vi "users Template Keys.vi"(6 "Current User Record":T1, 7 "Edit sxUsername (\"\")":string, 8 "error in (no error)":errorcluster, 9 "Copy? (f)":bool, 10 "Edit? (f)":bool, 11 "Connection Refnum":T2) -> (0 "error out":errorcluster, 1 "Template Keys":T3, 3 "Connection Refnum":T2)   [LabVIEW 2011]
uses:
  ITK EXT/utils/keyedarr.llb/Keyed Array.ctl
  Summitek EXT/ODBC/SQL Controls/Connection Refnum.ctl
  server/database/Users/User Record.ctl
  ITK EXT/utils/strutil.llb/Case Matching.ctl
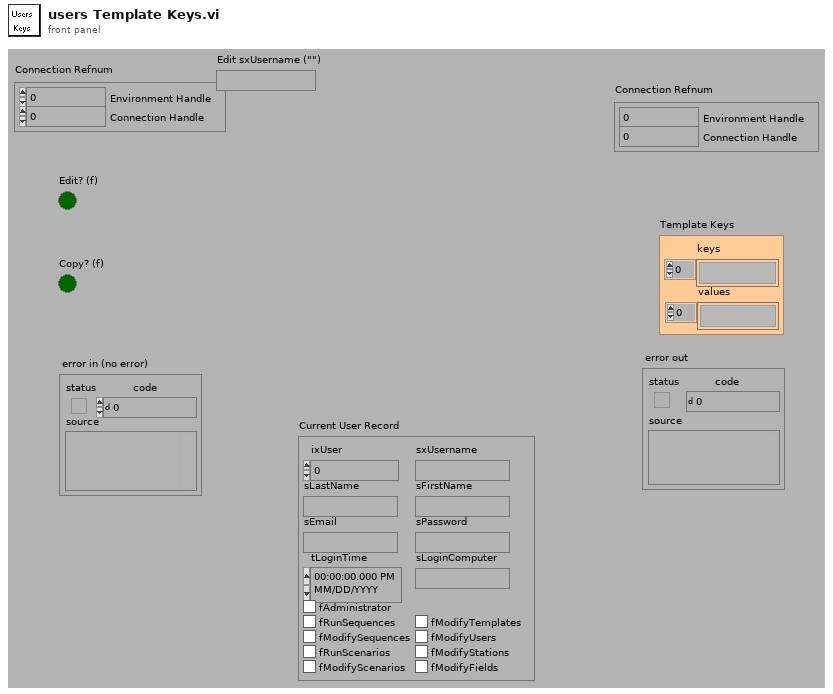
[diagram p1: front panel]
types:
  T1 = typedef "User Record.ctl" = cluster{"ixUser":i32, "sxUsername":string, "sLastName":string, "sFirstName":string, "sEmail":string, "sPassword":string, "tLoginTime":timestamp, "sLoginComputer":string, "fAdministrator":bool, "fRunSequences":bool, "fModifySequences":bool, "fRunScenarios":bool, "fModifyScenarios":bool, "fModifyTemplates":bool, "fModifyUsers":bool, "fModifyStations":bool, "fModifyFields":bool}
  T2 = typedef "Connection Refnum.ctl" = cluster{"Environment Handle":i32, "Connection Handle":i32}
  T3 = typedef "Keyed Array.ctl" = cluster{"keys":string[], "values":string[]}
  T4 = typedef "Authorization Data.ctl" = cluster{"Valid":bool, "Seats":i32, "Expire Time":timestamp, "Last Access Time":timestamp, "Product ID":string, "Hardware ID":string, "Spartan Serial Number":string, "Feature":cluster{"#attributes":cluster{"Name":string, "Value":string}}[]}
  T5 = typedef "Case Matching.ctl" = enum16{"a != A", "a == A", "system"}
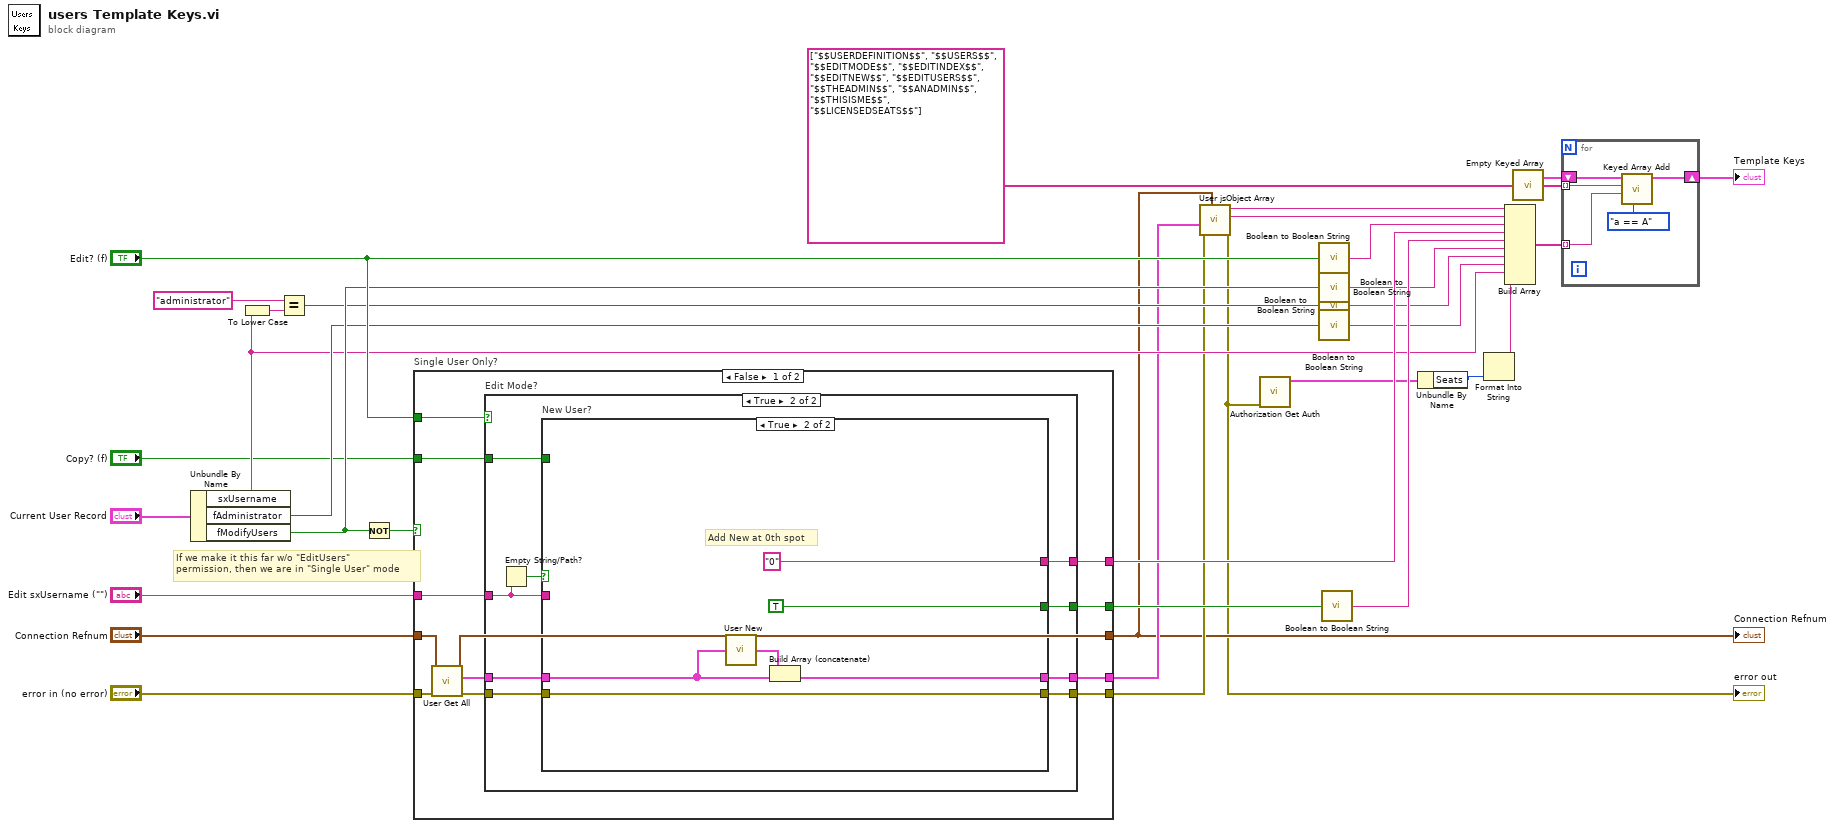
[diagram p0: block diagram]
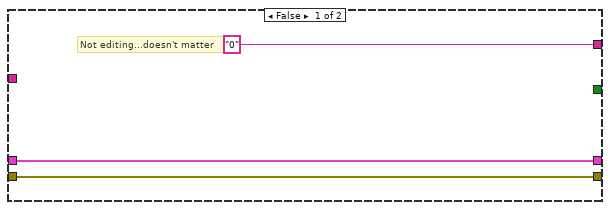
[diagram p2: hidden frame]
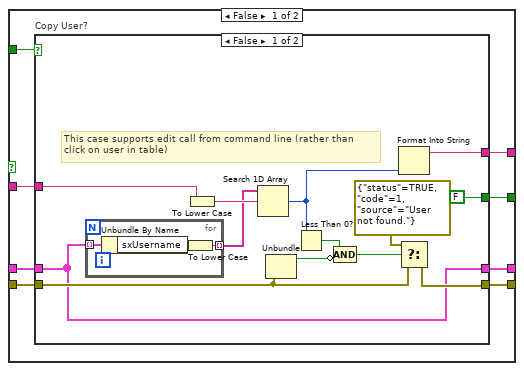
[diagram p3: hidden frame]
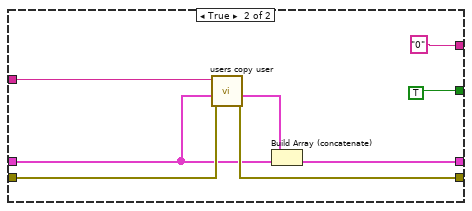
[diagram p4: hidden frame]
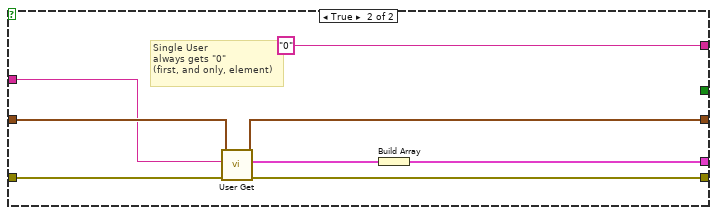
[diagram p5: hidden frame]
diagram:
  # "If we make it this far w/o \"EditUsers\"\npermission, then we are in \"Single User\" mode"
  n1 = Unbundle By Name("Current User Record") -> ("sxUsername"=w11:string, "fAdministrator"=w17:bool, "fModifyUsers"=w19:bool)
  n2 = To Lower Case(string=w11) -> (all lower case string=w15:string)
  n3 = Equal?(x="administrator", y=w15) -> (x = y?=w12:bool)
  n4 = Not(x=w19) -> (.not. x?=w25:bool)
  n5 = case "Single User Only?" shown="False" w25 {
    tunnel: "Connection Refnum" -> [w45 w99]
    tunnel: "error in (no error)" -> [w44 w102]
    tunnel: [w40 w103] -> w6
    tunnel: [w38 w101] -> w7
    tunnel: [w43 w98] -> w3
    tunnel: "Edit sxUsername (\"\")" -> [w36 w97]
    tunnel: [w37 "0"] -> w23
    tunnel: "Edit? (f)" -> [w41 _]
    tunnel: [w35 _] -> w20
    tunnel: "Copy? (f)" -> [w34 _]
    frame False {
      n6 = call "User Get All.vi"("error in (no error)"=w44, "Connection Refnum"=w45) -> ("error out"=w39:errorcluster, "User Records"=w42:T1[], "Connection Refnum"=w43:T2)  [unwired: 2 in, 5 out]
      n7 = case "Edit Mode?" shown="True" w41 {
        tunnel: w42 -> [w48 w57]
        tunnel: [w48 w53] -> w40
        tunnel: w39 -> [w47 w55]
        tunnel: [w47 w54] -> w38
        tunnel: ["0" w52] -> w37
        tunnel: w36 -> [_ w51]
        tunnel: [_ w50] -> w35
        tunnel: w34 -> [_ w49]
        frame False {
          # "Not editing...doesn't matter"
        }
        frame True {
          n8 = Empty String/Path?(string/path=w51) -> (empty?=w56:bool)
          n9 = case "New User?" shown="True" w56 {
            tunnel: w57 -> [w64 w90]
            tunnel: w55 -> [w61 w95]
            tunnel: [w62 w95] -> w54
            tunnel: [w58 w93] -> w53
            tunnel: [w63 "0"] -> w52
            tunnel: w51 -> [w65 _]
            tunnel: [w59 TRUE] -> w50
            tunnel: w49 -> [w60 _]
            frame False {
              n10 = case "Copy User?" shown="False" w60 {
                tunnel: w65 -> [w76 w83]
                tunnel: w64 -> [w66 w82]
                tunnel: [w74 "0"] -> w63
                tunnel: [w73 w86] -> w62
                tunnel: w61 -> [w72 w87]
                tunnel: [FALSE TRUE] -> w59
                tunnel: [w66 w84] -> w58
                frame False {
                  # "This case supports edit call from command line (rather than\nclick on user in table)"
                  n11 = for {
                    tunnel: w66 -> [w81] mode=indexing
                    tunnel: [w79] -> w77 mode=indexing
                    n12 = Unbundle By Name(w81) -> ("sxUsername"=w80:string)
                    n13 = To Lower Case(string=w80) -> (all lower case string=w79:string)
                  }
                  n14 = To Lower Case(string=w76) -> (all lower case string=w78:string)
                  n15 = Search 1D Array(1D array=w77, element=w78) -> (index of element=w75:i32)  [unwired: 1 out]
                  n16 = Unbundle(w72) -> ("status"=w71:bool)  [unwired: 2 out]
                  n17 = Less Than 0?(x=w75) -> (x < 0?=w70:bool)
                  n18 = Compound Arithmetic op=AND(w70, invert w71) -> (w69:bool)
                  n19 = Format Into String(w75) -> (resulting string=w74:string)  [unwired: 3 in, 1 out]
                  n20 = Select(t=errorcluster {"status"=TRUE, "code"=1, "source"="User not found."}, s=w69, f=w72) -> (s? t:f=w73:errorcluster)
                }
                frame True {
                  n21 = call "users copy user.vi"("error in (no error)"=w87, "All Users (empty)"=w82, "sxUsername (\"\")"=w83) -> ("error out"=w86:errorcluster, "User Information"=w85:T1)  [unwired: 7 out]
                  n22 = Build Array (concatenate)(w85, w82) -> (w84:T1[])
                }
              }
            }
            frame True {
              # "Add New at 0th spot"
              n23 = call "User New.vi"("Existing User Records (empty)"=w90) -> ("Default New User"=w94:T1)
              n24 = Build Array (concatenate)(w94, w90) -> (w93:T1[])
            }
          }
        }
      }
    }
    frame True {
      # "Single User \nalways gets \"0\"\n(first, and only, element)"
      n25 = call "User Get.vi"("error in (no error)"=w102, "sxUsername (\"\")"=w97, "Connection Refnum"=w99) -> ("error out"=w101:errorcluster, "User"=w100:T1, "Connection Refnum"=w98:T2)  [unwired: 6 out]
      n26 = Build Array(w100) -> (w103:T1[])
    }
  }
  "Connection Refnum" <- w3
  n27 = call "User jsObject Array.vi"("DB Connection Ref"=w3, "error in (no error)"=w7, "USERS (empty)"=w6) -> ("error out"=w1:errorcluster, "Users jsObject Array"=w5:string, "User jsObject Definition"=w4:string)  [unwired: 3 in, 3 out]
  "error out" <- w1
  n28 = call "Authorization Get Auth.vi"("error in (no error)"=w1) -> ("Authorization"=w2:T4)  [unwired: 9 in, 1 out]
  n29 = call "Boolean to Boolean String.vi"("Boolean"="Edit? (f)") -> ("Boolean string"=w27:string)  [unwired: 1 in]
  n30 = call "Boolean to Boolean String.vi"("Boolean"=w19) -> ("Boolean string"=w18:string)  [unwired: 1 in]
  n31 = call "Boolean to Boolean String.vi"("Boolean"=w12) -> ("Boolean string"=w13:string)  [unwired: 1 in]
  n32 = call "Boolean to Boolean String.vi"("Boolean"=w17) -> ("Boolean string"=w16:string)  [unwired: 1 in]
  n33 = call "Boolean to Boolean String.vi"("Boolean"=w20) -> ("Boolean string"=w21:string)  [unwired: 1 in]
  n34 = Unbundle By Name(w2) -> ("Seats"=w10:i32)
  n35 = Format Into String(w10) -> (resulting string=w9:string)  [unwired: 3 in, 1 out]
  n36 = Build Array(w4, w5, w27, w23, w21, w18, w13, w16, w11, w9) -> (w30:string[])
  n37 = call "Empty Keyed Array.vi"() -> ("empty keyed array"=w33:T3)  [unwired: 3 out]
  n38 = for {
    shift-right: [w105] -> w31
    shift-left: w33 -> [w107]
    tunnel: string[] ["$$USERDEFINITION$$", "$$USERS$$", "$$EDITMODE$$", "$$EDITINDEX$$", "$$EDITNEW$$", "$$EDITUSERS$$", "$$THEADMIN$$", "$$ANADMIN$$", "$$THISISME$$", "$$LICENSEDSEATS$$"] -> [w106] mode=indexing
    tunnel: w30 -> [w104] mode=indexing
    n39 = call "Keyed Array Add.vi"("case matching (sensitive)"=Case_Matching."a == A", "value"=w104, "key"=w106, "array in"=w107) -> ("array out"=w105:T3)  [unwired: 3 out]
  }
  "Template Keys" <- w31
